vi "RT Main-Core_Process.vi"   [LabVIEW 2015, in "RT Main-Core.lvclass"]
uses:
  RT Main-Core.lvclass
  source/actor/Message/Base/FTW-Message.lvclass
  source/actor/Instance/FTW-ActorInstance.lvclass/FTW-ActorInstance.ctl
  source/actor/JobSequencer/FTW-SEQ-Current.vi
  source/actor/Instance/FTW-ActorInstance.lvclass
  source/actor/Message/Request/FTW-Message-IncomingRequest.lvclass
  source/actor/Ether/FTW-Ether.lvclass
types:
  T1 = cluster{"Incoming Requests":refnum<event-registration>, "Local Messages":refnum<event-registration>, "Some Subscription":refnum<event-registration>}
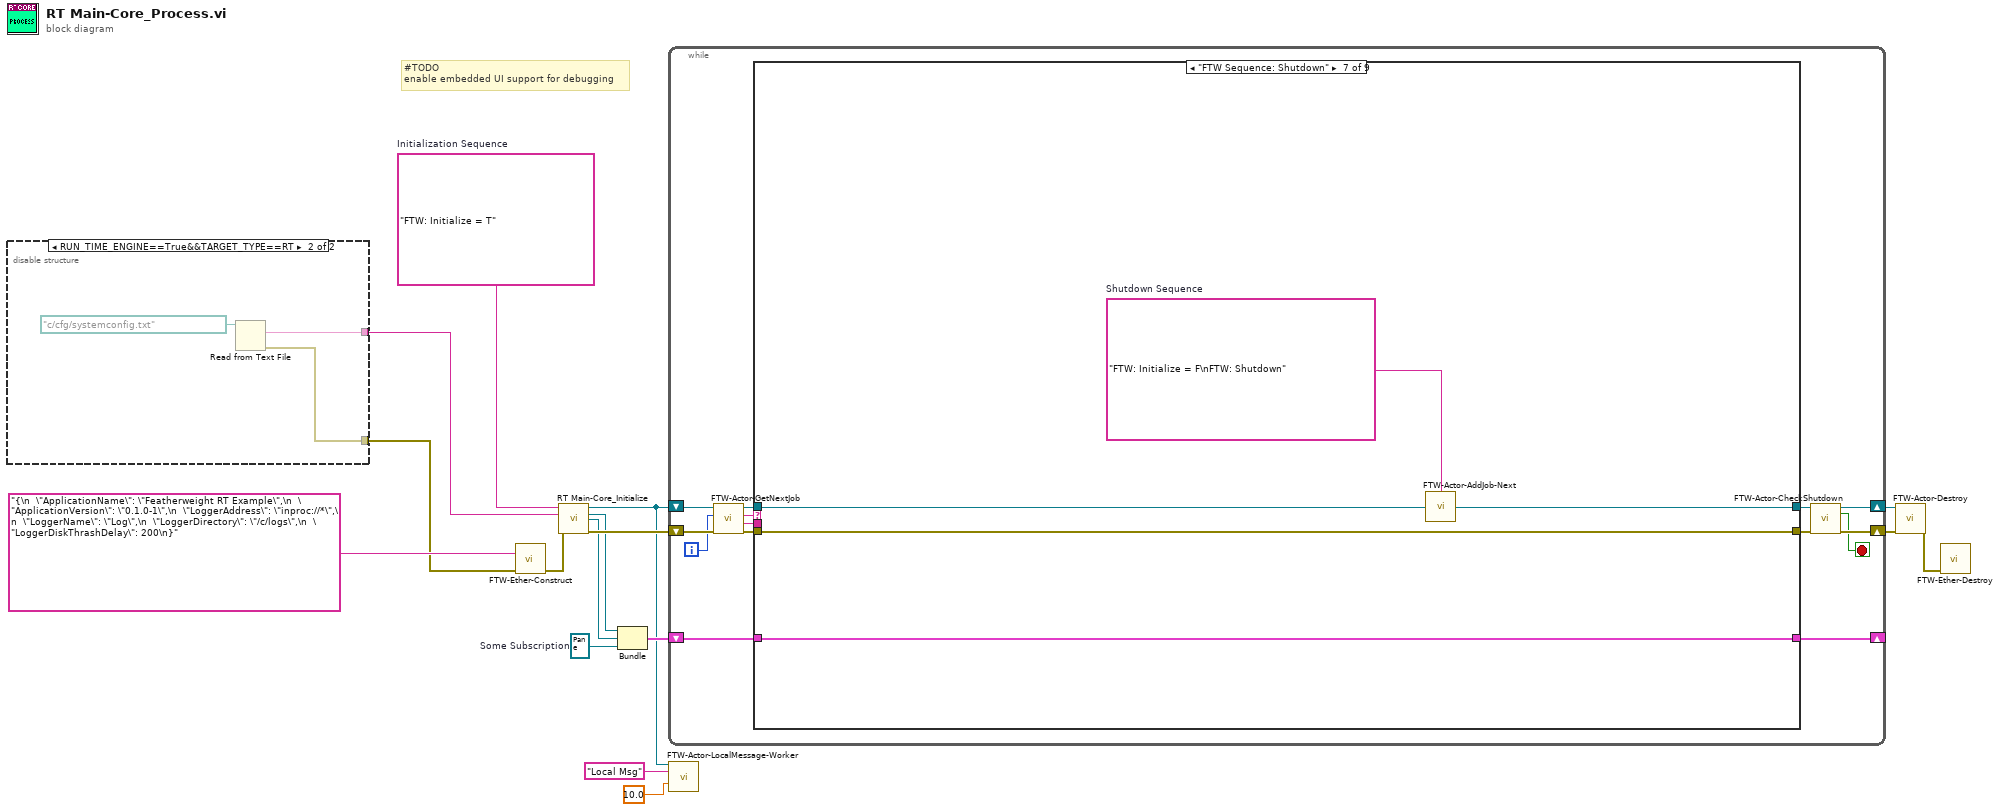
[diagram p0: block diagram]
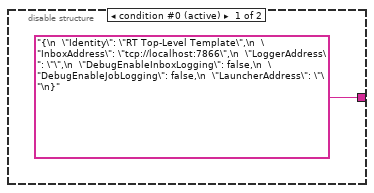
[diagram p2: hidden frame]
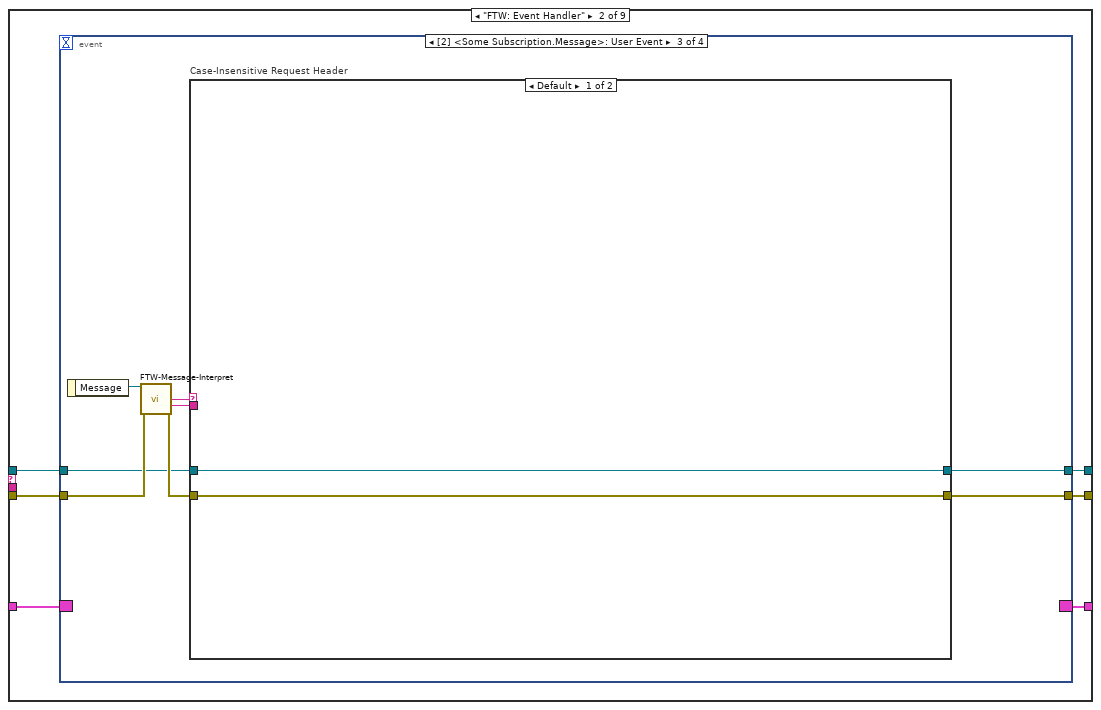
[diagram p4: hidden frame]
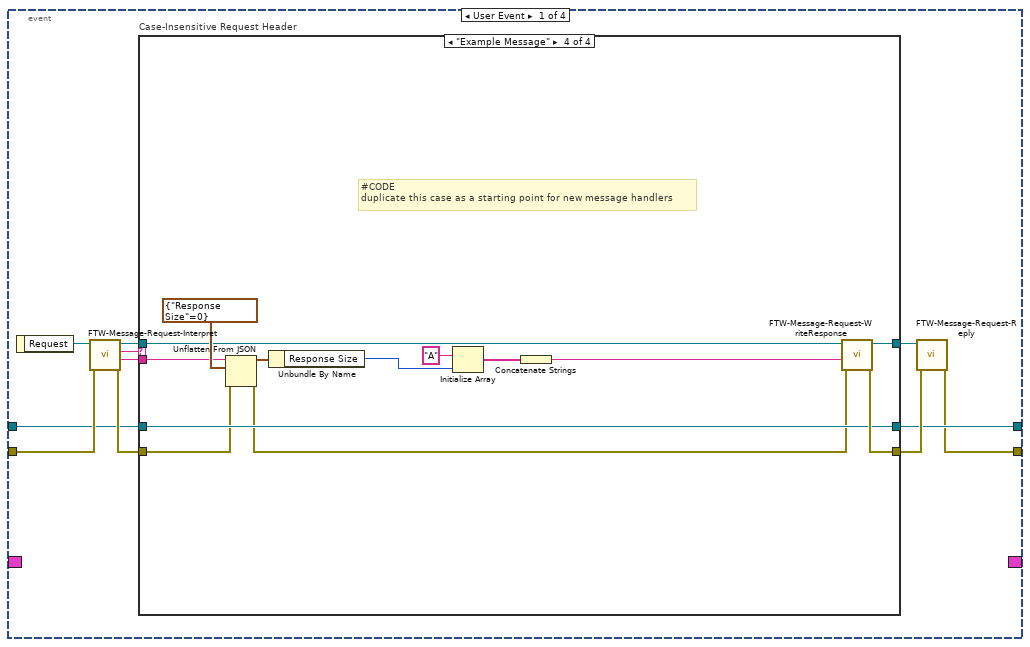
[diagram p5: hidden frame]
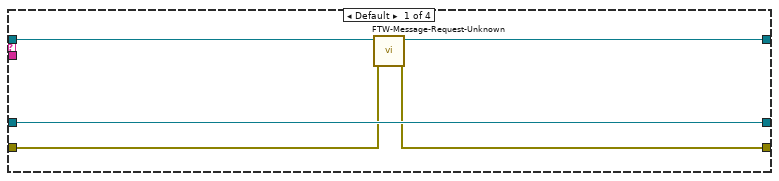
[diagram p6: hidden frame]
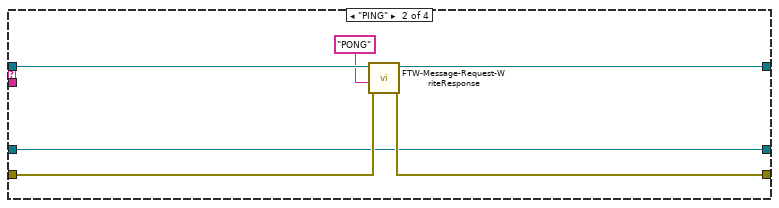
[diagram p7: hidden frame]
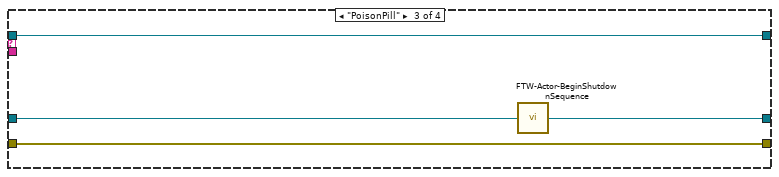
[diagram p8: hidden frame]
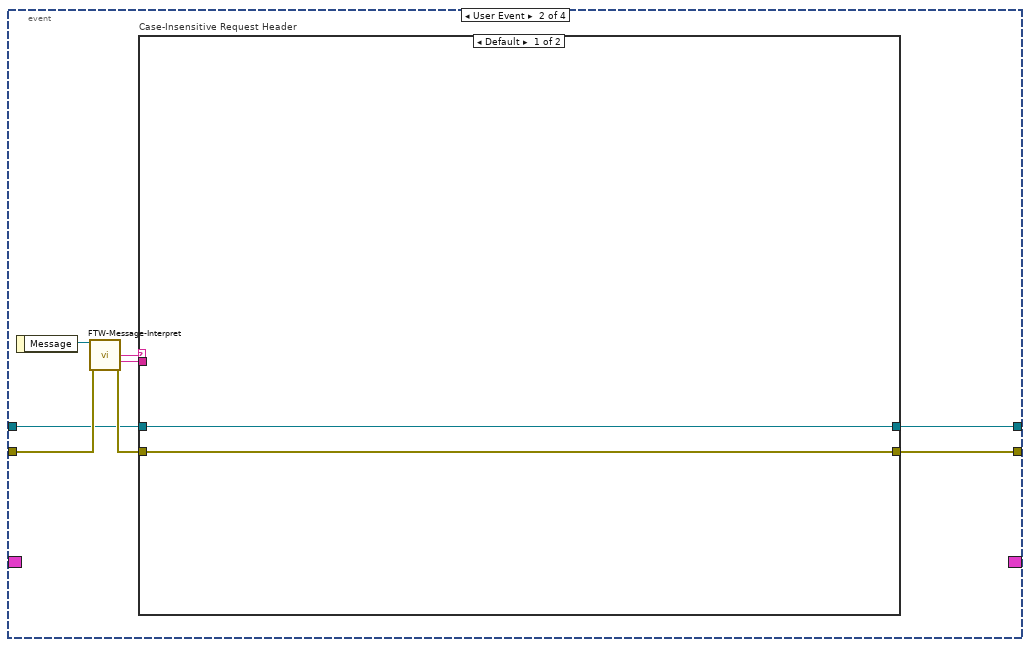
[diagram p9: hidden frame]
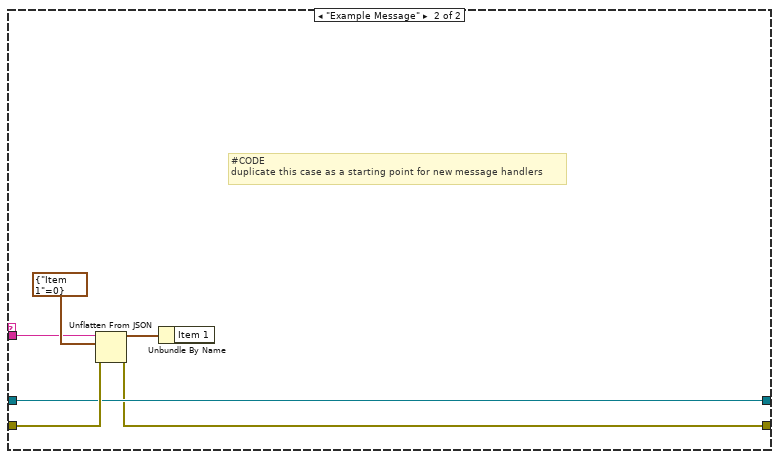
[diagram p10: hidden frame]
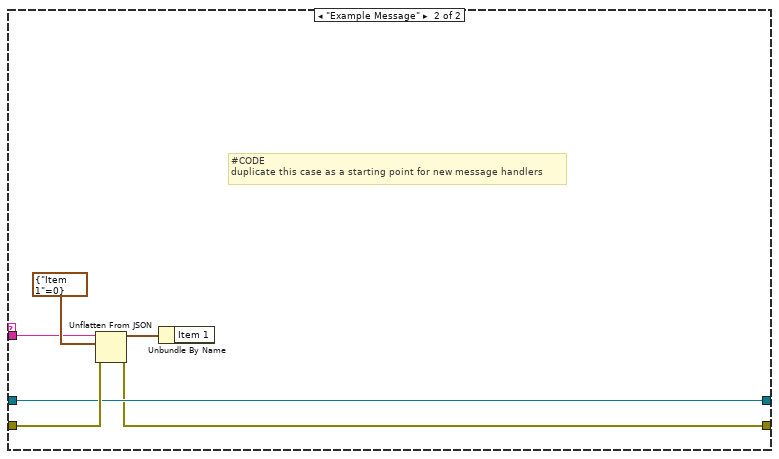
[diagram p11: hidden frame]
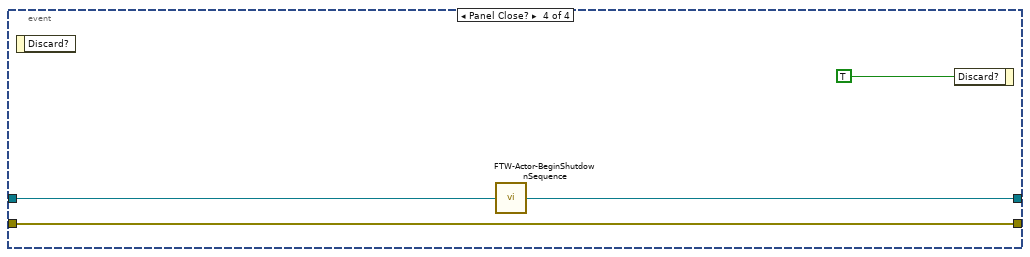
[diagram p12: hidden frame]
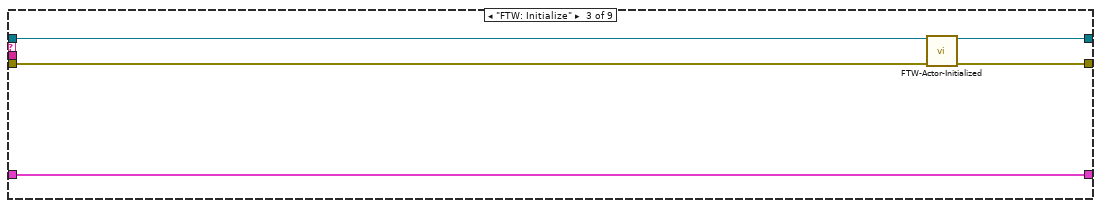
[diagram p13: hidden frame]
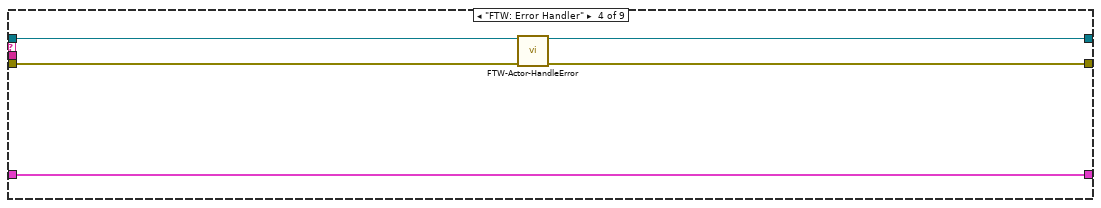
[diagram p14: hidden frame]
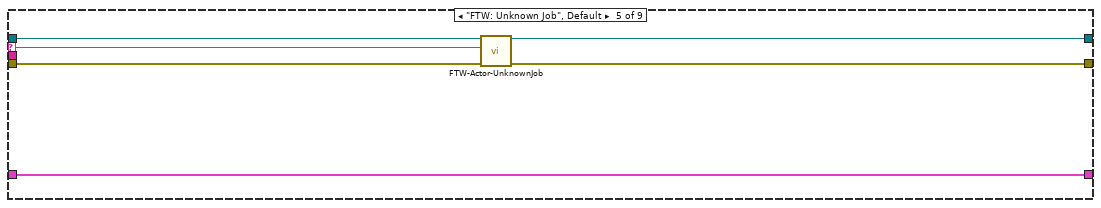
[diagram p15: hidden frame]
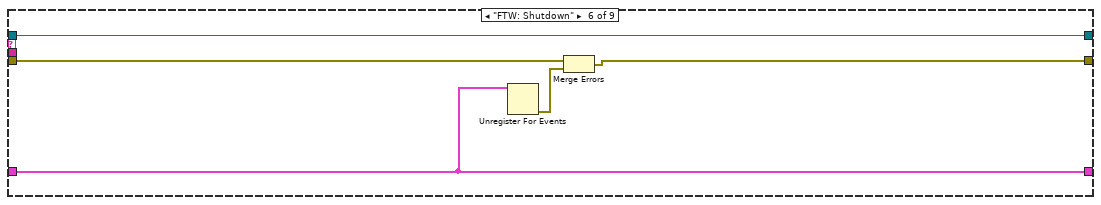
[diagram p16: hidden frame]
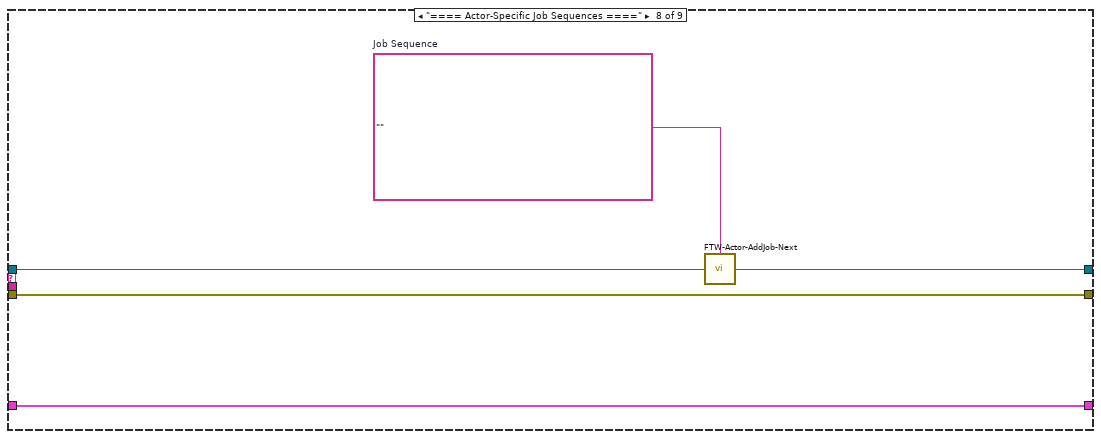
[diagram p17: hidden frame]
diagram:
  w10 = refnum<event-registration> refnum  # Some Subscription
  w2 = "FTW: Initialize = T"  # Initialization Sequence
  # "#TODO\nenable embedded UI support for debugging"
  n1 = disable-structure shown="RUN_TIME_ENGINE==True&&TARGET_TYPE==RT" {
    disable-tunnel: ["{\n  \"Identity\": \"RT Top-Level Template\",\n  \"InboxAddress\": \"tcp://localhost:7866\",\n  \"LoggerAddress\": \"\",\n  \"DebugEnableInboxLogging\": false,\n  \"DebugEnableJobLogging\": false,\n  \"LauncherAddress\": \"\"\n}" ("FTW Actor Instance Configuration") w19] -> w3
    disable-tunnel: [_ w18] -> w1
    frame condition #0 (active) {
    }
    frame condition #1 {
      n2 = Read from Text File(file (use dialog)=path "c:/cfg/systemconfig.txt") -> (text=w19:string, error out=w18:errorcluster)  [unwired: 3 in, 2 out]
    }
  }
  n3 = call "FTW-Ether-Construct.vi"("FTW Ether Configuration"="{\n  \"ApplicationName\": \"Featherweight RT Example\",\n  \"ApplicationVersion\": \"0.1.0-1\",\n  \"LoggerAddress\": \"inproc://*\",\n  \"LoggerName\": \"Log\",\n  \"LoggerDirectory\": \"/c/logs\",\n  \"LoggerDiskThrashDelay\": 200\n}", "error in"=w1) -> ("error out"=w9:errorcluster)  [unwired: 13 in]
  n4 = call "RT Main-Core_Initialize.vi"("Initialization Sequence"=w2, "FTW Actor Instance Configuration"=w3, "error in (no error)"=w9) -> ("Actor Template-Core out"=w6:refnum<class "RT Main-Core.lvclass">, "Incoming Requests"=w11:refnum<event-registration>, "Local Messages"=w7:refnum<event-registration>, "error out"=w13:errorcluster)  [unwired: 9 in]
  n5 = Bundle("Incoming Requests"=w11, "Local Messages"=w7, "Some Subscription"=w10) -> (w12:T1)  [unwired: 1 in]
  n6 = while {
    shift-right: [w24] -> w15
    shift-left: w13 -> [w31]
    shift-right: [w21] -> _
    shift-left: w12 -> [w34]
    shift-right: [w26] -> w16
    shift-left: w6 -> [w33]
    i -> [w22]
    stop <- w23 stop-if-true
    n7 = call "FTW-Actor-GetNextJob.vi"("error in"=w31, "Jobs Performed"=w22, "FTW Actor Instance"=w33) -> ("error out"=w30:errorcluster, "Job Data"=w28:string, "Job Name"=w29:string, "FTW Actor Instance out"=w32:refnum<class "RT Main-Core.lvclass">)  [unwired: 5 in]
    n8 = case shown="\"FTW Sequence: Shutdown\"" w29 {
      selector: w29 -> [_ _ _ _ w129 _ _ _ _]
      tunnel: [w36 w43 w119 w124 w132 w138 w143 w148 w152] -> w25
      tunnel: w30 -> [w36 w42 w122 w126 w133 w139 w143 w148 w152]
      tunnel: w34 -> [w37 w38 w123 w128 w134 w135 w144 w149 w151]
      tunnel: [w37 w41 w123 w128 w134 w135 w144 w149 w151] -> w21
      tunnel: w28 -> [_ _ _ _ _ _ _ _ _]
      tunnel: [w35 w40 w120 w125 w130 w136 w141 w146 w150] -> w27
      tunnel: w32 -> [w35 w39 w121 w127 w131 w136 w142 w147 w150]
      frame "==== Featherweight Framework Jobs ====" {
      }
      frame "FTW: Event Handler" {
        n9 = event shown="[2] <Some Subscription.Message>: User Event" {
          selector: w38 -> [_ _ _ _]
          dyn-events: [_ _ _ _] -> w41
          timeout: _ -> [_ _ _ _]
          tunnel: [w46 w87 w103 w117] -> w43
          tunnel: w42 -> [w52 w88 w104 w117]
          tunnel: [w50 w86 w102 w115] -> w40
          tunnel: w39 -> [w49 w85 w101 w116]
          event User Event {
            n10 = event-data() -> ("Request"=w53:refnum<class "FTW-Message-IncomingRequest.lvclass">)  [unwired: 1 in]
            n11 = call "FTW-Message-Request-Interpret.vi"("error in"=w52, "FTW Incoming Request"=w53) -> ("error out"=w54:errorcluster, "Request Body"=w44:string, "Request Header"=w48:string, "FTW Incoming Request out"=w47:refnum<class "FTW-Message-IncomingRequest.lvclass">)  [unwired: 6 in]
            n12 = case "Case-Insensitive Request Header" shown="\"Example Message\"" w48 {
              tunnel: [w57 w63 w68 w82] -> w51
              tunnel: w54 -> [w58 w64 w68 w70]
              tunnel: [w59 w62 w69 w80] -> w50
              tunnel: w49 -> [w59 w62 w67 w80]
              tunnel: w47 -> [w56 w65 w66 w72]
              tunnel: [w55 w61 w66 w81] -> w45
              tunnel: w44 -> [_ _ _ w71]
              frame Default {
                n13 = call "FTW-Message-Request-Unknown.vi"("error in"=w58, "FTW Incoming Request"=w56) -> ("error out"=w57:errorcluster, "FTW Incoming Request Out"=w55:refnum<class "FTW-Message-IncomingRequest.lvclass">)  [unwired: 8 in]
              }
              frame "PING" {
                n14 = call "FTW-Message-Request-WriteResponse.vi"("error in"=w64, "Response Body"="PONG" ("Response Header"), "FTW Incoming Request"=w65) -> ("error out"=w63:errorcluster, "FTW Incoming Request out"=w61:refnum<class "FTW-Message-IncomingRequest.lvclass">)  [unwired: 7 in]
              }
              frame "PoisonPill" {
                n15 = call "FTW-Actor-BeginShutdownSequence.vi"("FTW Actor Instance"=w67) -> ("FTW Actor Instance out"=w69:refnum<class "RT Main-Core.lvclass">)  [unwired: 3 in]
              }
              frame "Example Message" {
                # "#CODE\nduplicate this case as a starting point for new message handlers"
                n16 = Unflatten From JSON(JSON string=w71, type and defaults=cluster{"Response Size":i32} {"Response Size"=0}, error in (no error)=w70) -> (value=w77:cluster{"Response Size":i32}, error out=w79:errorcluster)  [unwired: 4 in]
                n17 = Unbundle By Name(w77) -> ("Response Size"=w76:i32)
                n18 = Initialize Array("A", w76) -> (w74:string[])
                n19 = Concatenate Strings(w74) -> (w73:string)
                n20 = call "FTW-Message-Request-WriteResponse.vi"("error in"=w79, "Response Body"=w73, "FTW Incoming Request"=w72) -> ("error out"=w82:errorcluster, "FTW Incoming Request out"=w81:refnum<class "FTW-Message-IncomingRequest.lvclass">)  [unwired: 7 in]
              }
            }
            n21 = call "FTW-Message-Request-Reply.vi"("FTW: Reply Error"=w51, "FTW Incoming Request"=w45) -> ("error out"=w46:errorcluster)  [unwired: 8 in, 1 out]
          }
          event User Event {
            n22 = event-data() -> ("Message"=w89:refnum<class "FTW-Message.lvclass">)  [unwired: 1 in]
            n23 = call-dynamic "FTW-Message-Interpret.vi"("FTW Message"=w89, "error in"=w88) -> ("Message Header"=w84:string, "Message Body"=w83:string, "error out"=w90:errorcluster)  [unwired: 9 in, 2 out]
            n24 = case "Case-Insensitive Request Header" shown="Default" w84 {
              tunnel: [w91 w96] -> w87
              tunnel: w90 -> [w91 w98]
              tunnel: [w92 w97] -> w86
              tunnel: w85 -> [w92 w97]
              tunnel: w83 -> [_ w93]
              frame Default {
              }
              frame "Example Message" {
                # "#CODE\nduplicate this case as a starting point for new message handlers"
                n25 = Unflatten From JSON(JSON string=w93, type and defaults=cluster{"Item 1":i32} {"Item 1"=0}, error in (no error)=w98) -> (value=w94:cluster{"Item 1":i32}, error out=w96:errorcluster)  [unwired: 4 in]
                n26 = Unbundle By Name(w94) -> ()  [unwired: 1 out]
              }
            }
          }
          event User Event {
            n27 = event-data() -> ("Message"=w105:refnum<class "FTW-Message.lvclass">)  [unwired: 1 in]
            n28 = call-dynamic "FTW-Message-Interpret.vi"("FTW Message"=w105, "error in"=w104) -> ("Message Header"=w100:string, "Message Body"=w99:string, "error out"=w106:errorcluster)  [unwired: 9 in, 2 out]
            n29 = case "Case-Insensitive Request Header" shown="Default" w100 {
              tunnel: [w107 w112] -> w103
              tunnel: w106 -> [w107 w114]
              tunnel: [w108 w113] -> w102
              tunnel: w101 -> [w108 w113]
              tunnel: w99 -> [_ w109]
              frame Default {
              }
              frame "Example Message" {
                # "#CODE\nduplicate this case as a starting point for new message handlers"
                n30 = Unflatten From JSON(JSON string=w109, type and defaults=cluster{"Item 1":i32} {"Item 1"=0}, error in (no error)=w114) -> (value=w110:cluster{"Item 1":i32}, error out=w112:errorcluster)  [unwired: 4 in]
                n31 = Unbundle By Name(w110) -> ()  [unwired: 1 out]
              }
            }
          }
          event Panel Close? {
            n32 = event-data() -> ()  [unwired: 1 in, 1 out]
            n33 = call "FTW-Actor-BeginShutdownSequence.vi"("FTW Actor Instance"=w116) -> ("FTW Actor Instance out"=w115:refnum<class "RT Main-Core.lvclass">)  [unwired: 3 in]
            n34 = event-data("Discard?"=TRUE) -> ()  [unwired: 1 in, 1 out]
          }
        }
      }
      frame "FTW: Initialize" {
        n35 = call-dynamic "FTW-Actor-Initialized.vi"("FTW Actor Instance"=w121, "error in"=w122) -> ("FTW Actor Instance out"=w120:refnum<class "RT Main-Core.lvclass">, "error out"=w119:errorcluster)  [unwired: 12 in]
      }
      frame "FTW: Error Handler" {
        n36 = call-dynamic "FTW-Actor-HandleError.vi"("FTW Actor Instance"=w127, "error in"=w126) -> ("FTW Actor Instance out"=w125:refnum<class "RT Main-Core.lvclass">, "error out"=w124:errorcluster)  [unwired: 10 in, 2 out]
      }
      frame "FTW: Unknown Job", Default {
        n37 = call-dynamic "FTW-Actor-UnknownJob.vi"("FTW Actor Instance"=w131, "Unknown Job"=w129, "error in"=w133) -> ("FTW Actor Instance out"=w130:refnum<class "RT Main-Core.lvclass">, "error out"=w132:errorcluster)  [unwired: 11 in]
      }
      frame "FTW: Shutdown" {
        n38 = Unregister For Events(event registration refnum=w135) -> (error out=w137:errorcluster)  [unwired: 1 in]
        n39 = Merge Errors(w139, w137) -> (w138:errorcluster)
      }
      frame "FTW Sequence: Shutdown" {
        w140 = "FTW: Initialize = F\nFTW: Shutdown"  # Shutdown Sequence
        n40 = call "FTW-Actor-AddJob-Next.vi"("Add Next in Job Queue"=w140, "FTW Actor Instance"=w142) -> ("FTW Actor Instance out"=w141:refnum<class "RT Main-Core.lvclass">)  [unwired: 2 in]
      }
      frame "==== Actor-Specific Job Sequences ====" {
        w145 = ""  # Job Sequence
        n41 = call "FTW-Actor-AddJob-Next.vi"("Add Next in Job Queue"=w145, "FTW Actor Instance"=w147) -> ("FTW Actor Instance out"=w146:refnum<class "RT Main-Core.lvclass">)  [unwired: 2 in]
      }
      frame "==== Actor-Specific Jobs ====" {
      }
    }
    n42 = call "FTW-Actor-CheckShutdown.vi"("FTW Actor Instance"=w27, "error in"=w25) -> ("FTW Actor Instance out"=w26:refnum<class "RT Main-Core.lvclass">, "Shutdown?"=w23:bool, "error out"=w24:errorcluster)  [unwired: 11 in]
  }
  n43 = call-dynamic "FTW-Actor-LocalMessage-Worker.vi"("FTW-ActorInstance In"=w6, "Message Header"="Local Msg", "Send Rate"=10.0) -> ()  [unwired: 13 in]
  n44 = call-dynamic "FTW-Actor-Destroy.vi"("FTW Actor Instance"=w16, "error in"=w15) -> ("error out"=w14:errorcluster)  [unwired: 13 in]
  n45 = call "FTW-Ether-Destroy.vi"("error in"=w14) -> ()  [unwired: 14 in, 1 out]
